vi "Gyro_Binary_Reader.vi"(8 "error in":errorcluster, 11 "file path (use dialog)":path) -> (0 "error out":errorcluster, 1 "Meta":T1={"# Pages"=0, "ODR"=0, "xlRange"=0, "gyroRange"=0, "id"=0, "Samplig Freq [Hz]"=9.980607627666451, "xlRange in g"=0.0, "gyroRange in dps"=0.0} {"id" format="%02d"; "xlRange" format="%02x"; "ODR" format="%02x"}, 2 "Angular Velocity":waveform(dbl)[](graph), 3 "Acceleration":waveform(dbl)[](graph))   [LabVIEW 2017]
uses:
  Controls/gyro_control_measurement_settings.ctl
panel:
  out "Battery Voltage":waveform(dbl)(graph)
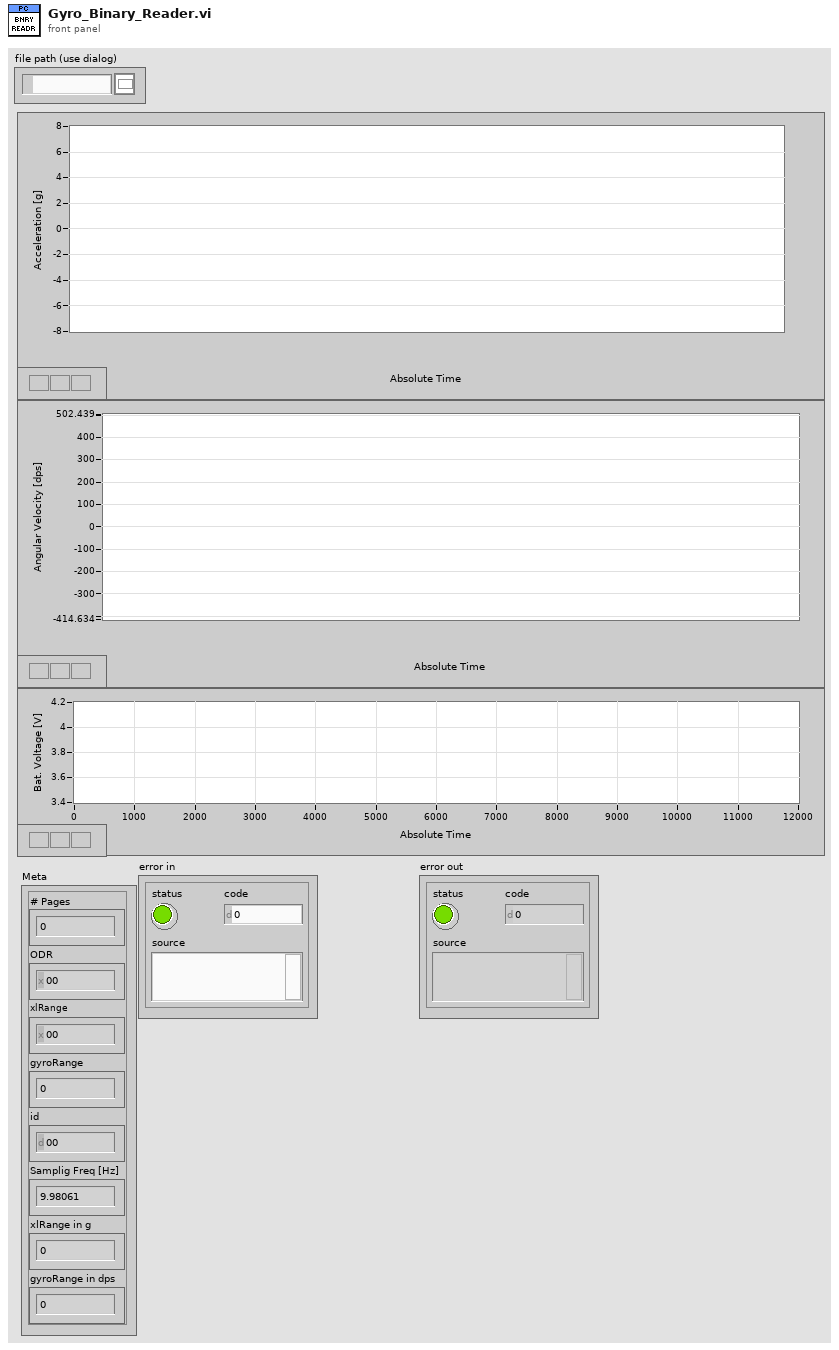
[diagram p1: front panel]
types:
  T1 = typedef "gyro_control_measurement_settings.ctl" = cluster{"# Pages":i32, "ODR":u8, "xlRange":u8, "gyroRange":u8, "id":u8, "Samplig Freq [Hz]":dbl, "xlRange in g":dbl, "gyroRange in dps":dbl}
  T2 = cluster{"Accel X":waveform(dbl), "Accel Y":waveform(dbl), "Accel Z":waveform(dbl), "Gyro X":waveform(dbl), "Gyro Y":waveform(dbl), "Gyro Z":waveform(dbl), "Battery":waveform(dbl)}
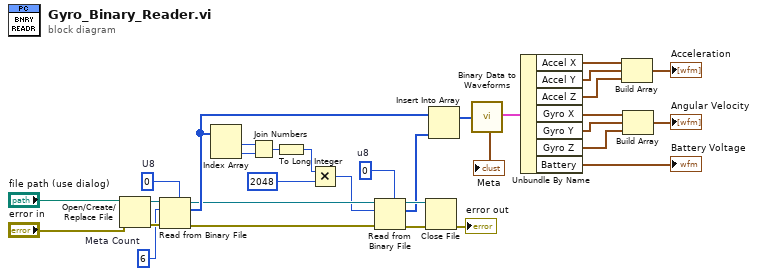
[diagram p0: block diagram]
diagram:
  w23 = u8 0  # u8
  w22 = u8 0  # U8
  w21 = 6  # Meta Count
  n1 = Open/Create/Replace File(file path (use dialog)="file path (use dialog)", error in="error in") -> (refnum out=w25:refnum<file>, error out=w24:errorcluster)  [unwired: 4 in, 1 out]
  n2 = Read from Binary File(5:w22, 8:w24, 10:w21, 11:w25) -> (0:w27:errorcluster, 2:w32:u8[], 3:w26:refnum<file>)  [unwired: 2 in, 1 out]
  n3 = Index Array(array=w32) -> (element #1=w30:u8, element #2=w31:u8)  [unwired: 2 in]
  n4 = Join Numbers(hi=w30, lo=w31) -> ((hi.lo)=w10:u16)
  n5 = To Long Integer(number=w10) -> (32bit integer=w9:i32)
  n6 = Multiply(x=w9, y=2048) -> (x*y=w7:i32)
  n7 = Read from Binary File(5:w23, 8:w27, 10:w7, 11:w26) -> (0:w28:errorcluster, 2:w11:u8[], 3:w29:refnum<file>)  [unwired: 2 in, 1 out]
  n8 = Close File(refnum=w29, error in=w28) -> (error out=→"error out":errorcluster)  [unwired: 1 out]
  n9 = Insert Into Array(array=w32, new element=w11) -> (w5:u8[])  [unwired: 1 in]
  n10 = call "Binary Data to Waveforms.vi"("Binary Data"=w5) -> ("Waveforms"=w4:T2, "Meta"=→"Meta":T1)
  n11 = Unbundle By Name(w4) -> ("Accel X"=w20:waveform(dbl), "Accel Y"=w18:waveform(dbl), "Accel Z"=w19:waveform(dbl), "Gyro X"=w16:waveform(dbl), "Gyro Y"=w17:waveform(dbl), "Gyro Z"=w15:waveform(dbl), "Battery"=→"Battery Voltage":waveform(dbl))
  n12 = Build Array(w20, w18, w19) -> (→"Acceleration":waveform(dbl)[])
  n13 = Build Array(w16, w17, w15) -> (→"Angular Velocity":waveform(dbl)[])
